vi "File Page - Init .NET Controls.vi"(7 "File Ctl Refs":T1, 8 "error in (no error)":errorcluster, 11 "Item Ref in":T11 format="%.0x") -> (0 "error out":errorcluster, 3 "Item Ref out":T11 format="%.0x")   [LabVIEW 2015, in "Waveform Data Logger System Explorer.lvlib"]
uses:
  Waveform Data Logger System Explorer.lvlib
  <vilib>/NI Veristand/Custom Device API/Custom Device Item Ref.ctl
  Types/File Ctl Refs.ctl
  Types/File - Spec Ctl Refs.ctl
  Types/File - Wfm Ctl Refs.ctl
  Types/File - Settings Ctl Refs.ctl
  Shared/Classes/Log File Specifications/Log File Specification/File Conflict Operation.ctl
  Types/File - Start Trig Ctl Refs.ctl
  Shared/Types/Start Trigger.ctl
  Shared/Types/Default Trigger.ctl
  Shared/Types/Digital Trigger.ctl
  Shared/Types/Analog Trigger.ctl
  Shared/Types/In Range Trigger.ctl
  Shared/Types/Value Change Trigger.ctl
  Shared/Types/Boolean Trigger.ctl
  Types/Single Node Browser Data.ctl
  <vilib>/NI Veristand/UI Controls/Single Node Browser/Single Node Browser Ref.ctl
  NationalInstruments.VeriStand.SystemStorageUI
  <vilib>/NI Veristand/UI Controls/Single Node Browser/Callback Type.ctl
  <vilib>/NI Veristand/UI Controls/Single Node Browser/Net Event Data.ctl
  <vilib>/NI Veristand/UI Controls/Single Node Browser/Net Event.ctl
  Types/File - Stop Trig Ctl Refs.ctl
  Shared/Types/Stop Trigger.ctl
  Types/File - Advanced Ctl Refs.ctl
  Types/Log Timestamps.ctl
  NationalInstruments.VeriStand.SystemStorage
  Shared/Globals/Property Strings.vi
  <vilib>/NI Veristand/Custom Device API/Get Item Property (Dependent Node Pointer).vi
  Shared/Waveform Data Logger Shared.lvlib
  <vilib>/NI VeriStand/Custom Device API/Custom Device API.lvlib
  <vilib>/NI VeriStand/Custom Device Tools/Custom Device Utility Library/Custom Device Utility Library.lvlib
  Shared/Classes/Log File Specifications/Log File Specification/Log File Specification.lvclass
  <vilib>/NI VeriStand/UI Controls/Single Node Browser/NI_VS UI Single Node Browser.lvlib
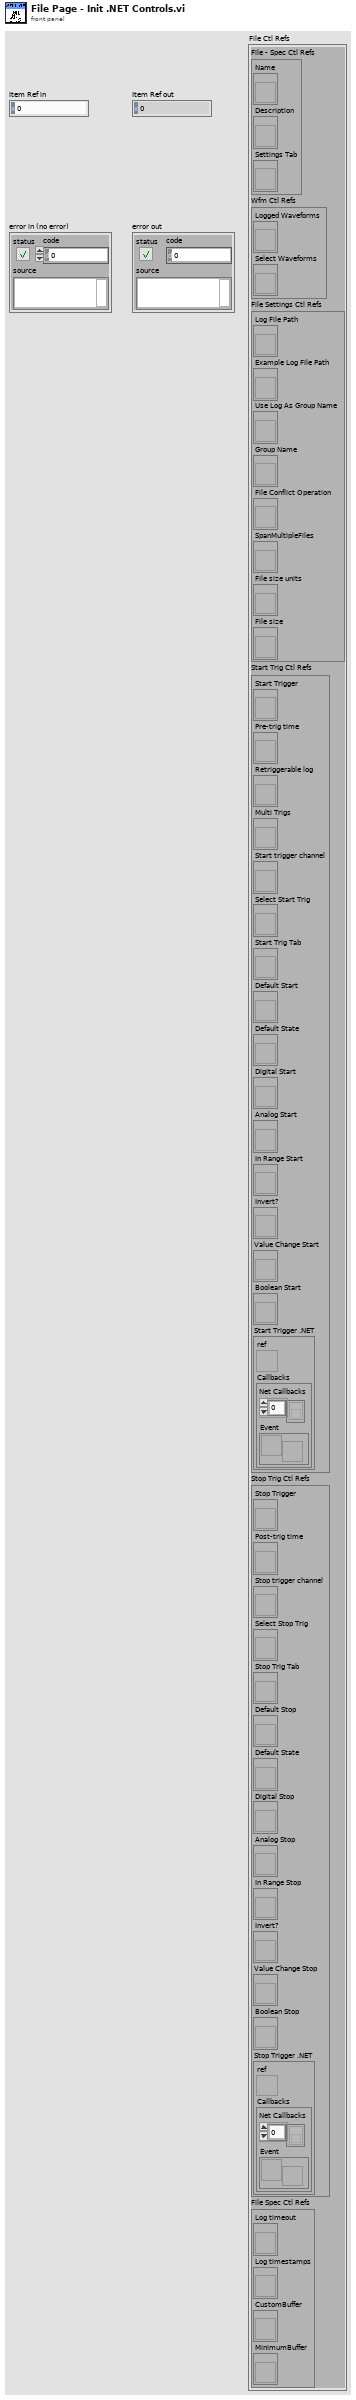
[diagram p1: front panel]
types:
  T1 = typedef "Waveform Data Logger System Explorer.lvlib/File Ctl Refs.ctl" = cluster{"File Spec Ctl Refs":T2, "Wfm Ctl Refs":T3, "File Settings Ctl Refs":T4, "Start Trig Ctl Refs":T5, "Stop Trig Ctl Refs":T9, "File Spec Ctl Refs":T10}
  T2 = typedef "Waveform Data Logger System Explorer.lvlib/File - Spec Ctl Refs.ctl" = cluster{"Name":refnum<vi>, "Description":refnum<vi>, "Settings Tab":refnum<vi>}
  T3 = typedef "Waveform Data Logger System Explorer.lvlib/File - Wfm Ctl Refs.ctl" = cluster{"Logged Waveforms":refnum<vi>, "Select Waveforms":refnum<vi>}
  T4 = typedef "Waveform Data Logger System Explorer.lvlib/File - Settings Ctl Refs.ctl" = cluster{"Log File Path":refnum<vi>, "Example Log File Path":refnum<vi>, "Use Log As Group Name":refnum<vi>, "Group Name":refnum<vi>, "File Conflict Operation":refnum<vi>, "SpanMultipleFiles":refnum<vi>, "File size units":refnum<vi>, "File size":refnum<vi>}
  T5 = typedef "Waveform Data Logger System Explorer.lvlib/File - Start Trig Ctl Refs.ctl" = cluster{"Start Trigger":refnum<vi>, "Pre-trig time":refnum<vi>, "Retriggerable log":refnum<vi>, "Multi Trigs":refnum<vi>, "Start trigger channel":refnum<vi>, "Select Start Trig":refnum<vi>, "Start Trig Tab":refnum<vi>, "Default Start":refnum<vi>, "Default State":refnum<vi>, "Digital Start":refnum<vi>, "Analog Start":refnum<vi>, "In Range Start":refnum<vi>, "Invert?":refnum<vi>, "Value Change Start":refnum<vi>, "Boolean Start":refnum<vi>, "Start Trigger .NET":T6}
  T6 = typedef "Waveform Data Logger System Explorer.lvlib/Single Node Browser Data.ctl" = cluster{"ref":T7, "Callbacks":T8}
  T7 = typedef "NI_VS UI Single Node Browser.lvlib/Single Node Browser Ref.ctl" = refnum<k24>
  T8 = typedef "NI_VS UI Single Node Browser.lvlib/Callback Type.ctl" = cluster{"Net Callbacks":refnum<k27>[], "Event":refnum<user-event>}
  T9 = typedef "Waveform Data Logger System Explorer.lvlib/File - Stop Trig Ctl Refs.ctl" = cluster{"Stop Trigger":refnum<vi>, "Post-trig time":refnum<vi>, "Stop trigger channel":refnum<vi>, "Select Stop Trig":refnum<vi>, "Stop Trig Tab":refnum<vi>, "Default Stop":refnum<vi>, "Default State":refnum<vi>, "Digital Stop":refnum<vi>, "Analog Stop":refnum<vi>, "In Range Stop":refnum<vi>, "Invert?":refnum<vi>, "Value Change Stop":refnum<vi>, "Boolean Stop":refnum<vi>, "Stop Trigger .NET":T6}
  T10 = typedef "Waveform Data Logger System Explorer.lvlib/File - Advanced Ctl Refs.ctl" = cluster{"Log timeout":refnum<vi>, "Log timestamps":refnum<vi>, "CustomBuffer":refnum<vi>, "MinimumBuffer":refnum<vi>}
  T11 = typedef "Custom Device API.lvlib/Custom Device Item Ref.ctl" = u64
  T12 = typedef "Custom Device API.lvlib/Custom Device Pointer.ctl" = refnum<k24>
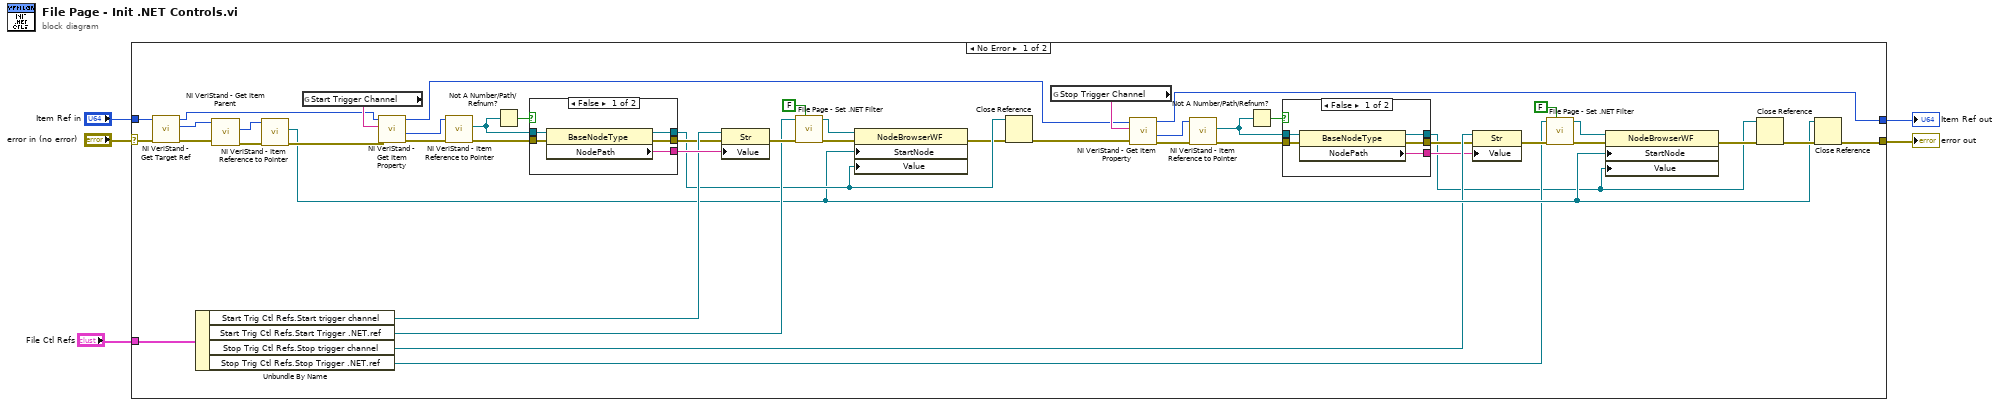
[diagram p0: block diagram]
diagram:
  n1 = case shown="No Error" "error in (no error)" {
    selector: "error in (no error)" -> [w42 w67]
    tunnel: [w15 w68] -> w5
    tunnel: [w21 w67] -> w4
    tunnel: "Item Ref in" -> [w41 w68]
    tunnel: "File Ctl Refs" -> [w52 _]
    frame No Error {
      n2 = call <vilib>:"NI VeriStand - Get Target Ref.vi"("error in"=w42, "Item Ref in"=w41) -> ("error out"=w40:errorcluster, "Target Ref"=w43:T11, "Item Ref out"=w18:T11)  [unwired: 6 in, 1 out]
      n3 = Unbundle By Name(w52) -> ("Start Trig Ctl Refs.Start trigger channel"=w45:refnum<vi>, "Start Trig Ctl Refs.Start Trigger .NET.ref"=w35:T7, "Stop Trig Ctl Refs.Stop trigger channel"=w20:refnum<vi>, "Stop Trig Ctl Refs.Stop Trigger .NET.ref"=w19:T7)
      n4 = call <vilib>:"NI VeriStand - Get Item Parent.vi"("error in (no error)"=w40, "Item Ref in"=w43) -> ("error out"=w39:errorcluster, "Parent Ref"=w44:T11)  [unwired: 6 in, 2 out]
      n5 = call <vilib>:"NI VeriStand - Item Reference to Pointer.vi"("error in (no error)"=w39, "Item Ref in"=w44) -> ("error out"=w38:errorcluster, "Node Pointer"=w22:T12)  [unwired: 6 in, 2 out]
      n6 = global read "Property Strings.vi" "Start Trigger Channel"() -> (w51:string)
      n7 = call-poly <vilib>:"NI VeriStand - Get Item Property.vi"("error in (no error)"=w38, "Property Name"=w51, "Item Ref in"=w18) -> ("error out"=w49:errorcluster, "Dependent Node Ref"=w17:T11, "Item Ref out"=w14:T11)  [unwired: 6 out]
      n8 = call <vilib>:"NI VeriStand - Item Reference to Pointer.vi"("error in (no error)"=w49, "Item Ref in"=w17) -> ("error out"=w48:errorcluster, "Node Pointer"=w13:T12)  [unwired: 6 in, 2 out]
      n9 = Not A Number/Path/Refnum?(number/path/refnum=w13) -> (NaN/Path/Refnum?=w12:bool)
      n10 = case shown="False" w12 {
        tunnel: w48 -> [w64 w65]
        tunnel: [w63 _] -> w47
        tunnel: [w62 w65] -> w37
        tunnel: [w61 w66] -> w31
        tunnel: w13 -> [w60 w66]
        frame False {
          n11 = property class="BaseNodeType"(reference=w60, error in=w64) -> (reference out=w61:T12, error out=w62:errorcluster, "NodePath"=w63:string)
        }
        frame True {
        }
      }
      n12 = property class="Str"(reference=w45, error in=w37, "Value"=w47) -> (error out=w36:errorcluster)  [unwired: 1 out]
      n13 = call "File Page - Set .NET Filter.vi"("Include Wfms?"=FALSE, "error in (no error)"=w36, "Trigger Control in"=w35) -> ("error out"=w33:errorcluster, "Trigger Control out"=w32:T7)  [unwired: 7 in]
      n14 = property class="NodeBrowserWF"(reference=w32, error in=w33, "StartNode"=w22, "Value"=w31) -> (error out=w30:errorcluster)  [unwired: 1 out]
      n15 = Close Reference(reference=w31, error in (no error)=w30) -> (error out=w29:errorcluster)
      n16 = global read "Property Strings.vi" "Stop Trigger Channel"() -> (w50:string)
      n17 = call-poly <vilib>:"NI VeriStand - Get Item Property.vi"("error in (no error)"=w29, "Property Name"=w50, "Item Ref in"=w14) -> ("error out"=w46:errorcluster, "Dependent Node Ref"=w16:T11, "Item Ref out"=w15:T11)  [unwired: 6 out]
      n18 = call <vilib>:"NI VeriStand - Item Reference to Pointer.vi"("error in (no error)"=w46, "Item Ref in"=w16) -> ("error out"=w6:errorcluster, "Node Pointer"=w7:T12)  [unwired: 6 in, 2 out]
      n19 = Not A Number/Path/Refnum?(number/path/refnum=w7) -> (NaN/Path/Refnum?=w11:bool)
      n20 = case shown="False" w11 {
        tunnel: w6 -> [w57 w58]
        tunnel: [w56 _] -> w10
        tunnel: [w55 w58] -> w9
        tunnel: [w54 w59] -> w8
        tunnel: w7 -> [w53 w59]
        frame False {
          n21 = property class="BaseNodeType"(reference=w53, error in=w57) -> (reference out=w54:T12, error out=w55:errorcluster, "NodePath"=w56:string)
        }
        frame True {
        }
      }
      n22 = property class="Str"(reference=w20, error in=w9, "Value"=w10) -> (error out=w24:errorcluster)  [unwired: 1 out]
      n23 = call "File Page - Set .NET Filter.vi"("Include Wfms?"=FALSE, "error in (no error)"=w24, "Trigger Control in"=w19) -> ("error out"=w26:errorcluster, "Trigger Control out"=w27:T7)  [unwired: 7 in]
      n24 = property class="NodeBrowserWF"(reference=w27, error in=w26, "StartNode"=w22, "Value"=w8) -> (error out=w28:errorcluster)  [unwired: 1 out]
      n25 = Close Reference(reference=w8, error in (no error)=w28) -> (error out=w23:errorcluster)
      n26 = Close Reference(reference=w22, error in (no error)=w23) -> (error out=w21:errorcluster)
    }
    frame Error {
    }
  }
  "error out" <- w4
  "Item Ref out" <- w5
